vi "Force Calibration Finished.vi"(8 "error in (no error)":errorcluster, 10 "Force calibratred values":cluster{"mean":dbl, "mean":dbl}, 11 "GUI in":refnum<class "GUI.lvclass">) -> (0 "error out":errorcluster, 3 "GUI out":refnum<class "GUI.lvclass">)   [LabVIEW 2020, in "GUI.lvlib" / "GUI.lvclass"]
uses:
  GUI.lvclass
  GUI.lvclass/GUI.ctl
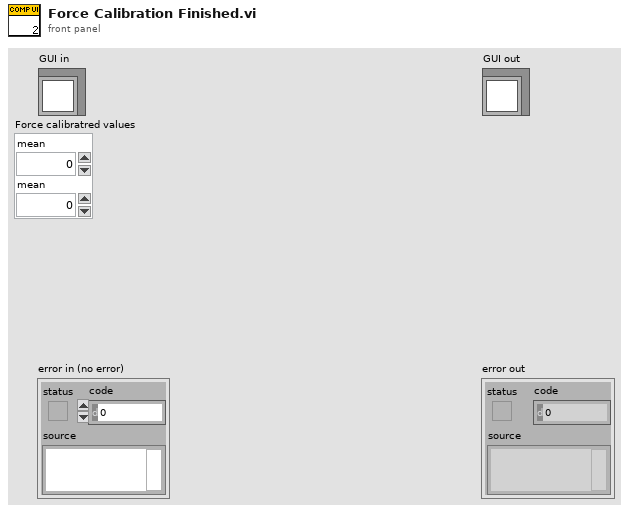
[diagram p1: front panel]
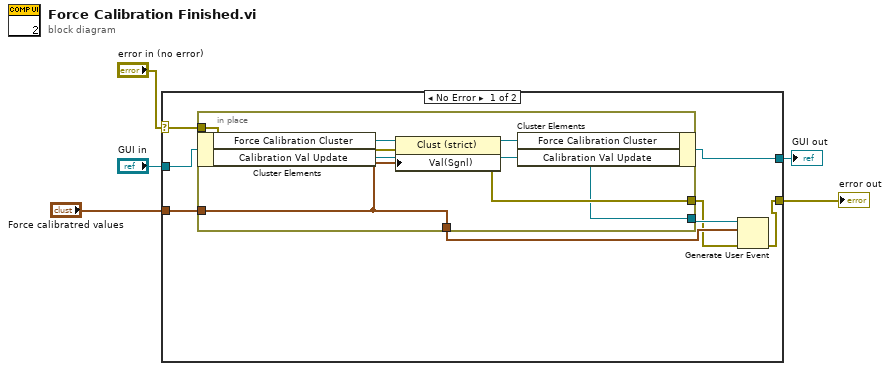
[diagram p0: block diagram]
diagram:
  n1 = case shown="No Error" "error in (no error)" {
    selector: "error in (no error)" -> [w11 w20]
    tunnel: "GUI in" -> [w13 w21]
    tunnel: "Force calibratred values" -> [w12 _]
    tunnel: [w10 w21] -> w2
    tunnel: [w6 w20] -> w1
    frame No Error {
      n2 = in-place {
        in-place-border: w12 -> [w14]
        in-place-border: w11 -> [w17]
        in-place-border: [w16] -> w7
        in-place-border: [w15] -> w9
        in-place-border: [w14] -> w8
        n3 = in-place-cluster #1(w13) -> ("Force Calibration Cluster"=w19:refnum<vi>, "Calibration Val Update"=w15:refnum<user-event>)
        n4 = property class="Clust (strict)"(reference=w19, error in=w17, "Val(Sgnl)"=w14) -> (reference out=w18:refnum<vi>, error out=w16:errorcluster)
        n5 = in-place-cluster #1("Force Calibration Cluster"=w18, "Calibration Val Update"=w15) -> (w10:refnum<class "GUI.lvclass">)
      }
      n6 = Generate User Event(user event=w9, event data cluster=w8, error in=w7) -> (error out=w6:errorcluster)  [unwired: 1 in, 1 out]
    }
    frame Error {
    }
  }
  "GUI out" <- w2
  "error out" <- w1
